vi "Position relative to InPlace.vi"(11 "InPlaceClusterNode in":refnum<vi>) -> (3 "Position":enum16{"Left", "Top", "Right", "Bottom"}(ring))   [LabVIEW 2023]
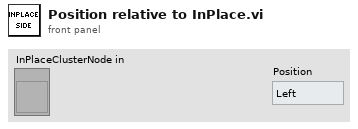
[diagram p1: front panel]
types:
  T1 = typedef "LVRectTypeDef.ctl" = cluster{"Left":i16, "Top":i16, "Right":i16, "Bottom":i16}
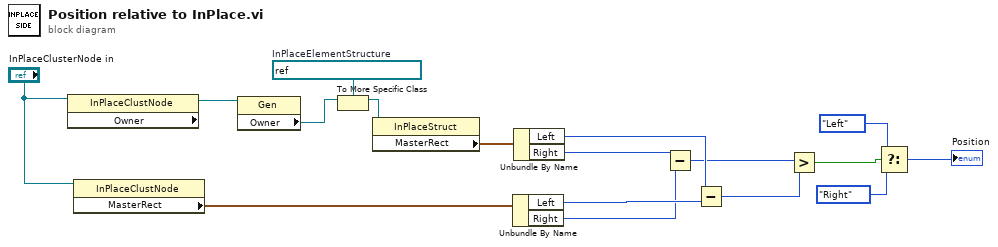
[diagram p0: block diagram]
diagram:
  w15 = refnum<vi> refnum  # InPlaceElementStructure
  n1 = property class="InPlaceClustNode"(reference="InPlaceClusterNode in") -> ("Owner"=w13:refnum<vi>)  [unwired: 1 in, 2 out]
  n2 = property class="InPlaceClustNode"(reference="InPlaceClusterNode in") -> ("MasterRect"=w12:T1)  [unwired: 1 in, 2 out]
  n3 = property class="Gen"(reference=w13) -> ("Owner"=w16:refnum<vi>)  [unwired: 1 in, 2 out]
  n4 = To More Specific Class(target class=w15, reference=w16) -> (specific class reference=w17:refnum<vi>)  [unwired: 1 in, 1 out]
  n5 = property class="InPlaceStruct"(reference=w17) -> ("MasterRect"=w11:T1)  [unwired: 1 in, 2 out]
  n6 = Unbundle By Name(w12) -> ("Left"=w10:i16, "Right"=w8:i16)
  n7 = Unbundle By Name(w11) -> ("Left"=w9:i16, "Right"=w7:i16)
  n8 = Subtract(x=w8, y=w7) -> (x-y=w6:i16)
  n9 = Subtract(x=w9, y=w10) -> (x-y=w5:i16)
  n10 = Greater?(x=w6, y=w5) -> (0:w4:bool)
  n11 = Select(t=enum16{"Left", "Top", "Right", "Bottom"}."Left" ("Position"), s=w4, f=enum16{"Left", "Top", "Right", "Bottom"}."Right" ("Position")) -> (s? t:f=→"Position":enum16{"Left", "Top", "Right", "Bottom"})
